vi "Unit test-Encoder triggering.vi"() -> ()   [LabVIEW 2017]
uses:
  Typedefs/Imaging Protocols enum.ctl
  Typedefs/Frame Size.ctl
  Typedefs/Logging queue element.ctl
  Peripherals Control/Pockels/Globals/gl_Pockels control globals.vi
  Typedefs/Acquired points count.ctl
panel:
  out "# of DO points":i32
  in  "Imaging Protocol":T1=enum."Live Imaging"
  out "Waveform Graph":dbl[](graph)
  out "Execution time (ms)":u32
  in  "AO high value":dbl(knob) scale=0.0..2.0
  in  "Start:More:Retriggerable (T)":bool=TRUE
  out "Loop":i32
  out "# of AO points":i32
  in  "stop":bool
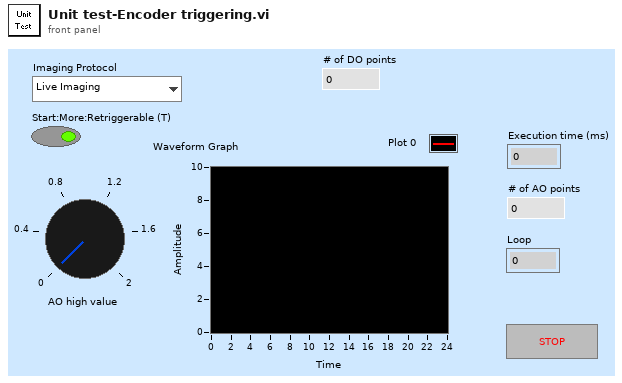
[diagram p1: front panel]
types:
  T1 = typedef "Imaging Protocols enum.ctl" = enum16{"AOL Z-Stack", "Motor Z Stack", "Functional Acquisition", "Single Plane Acquisition", "Volume Acquisition", "Live Imaging", "Live Plane Imaging", "Live Volume Imaging"}
  T2 = typedef "Logging queue element.ctl" = cluster{"Imaging Protocol":T1, "Number of Trials":u16, "Frame Size":T3, "# Averaged frames":u16, "Dwell time (us)":dbl, "Index of Z-plane":i32, "Timelapse?":bool, "Logging process is active":bool, "Speed logging enabled":bool, "tdms file ref":refnum<k34>, "path":path, "Trial Number":i32, "Expected # points acquired":bool, "Manually stopped":bool, "Ch0 data":u32[], "Ch1 data":u32[], "Ref Data":u32[], "Last trial":bool, "Ref Dwell time (us)":dbl, "# Ref Averaged frames":u16, "Ref X Length":u16, "Ref Y Length":u16, "Points acquired":T4}
  T3 = typedef "Frame Size.ctl" = u16
  T4 = typedef "Acquired points count.ctl" = cluster{"Ch0 last trial":u64, "Ch1 last trial":u64, "All trials":u64}
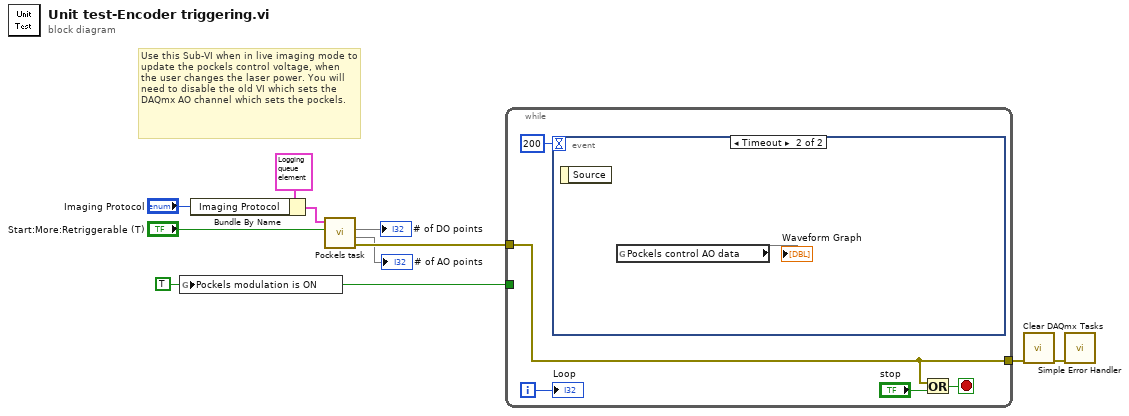
[diagram p0: block diagram]
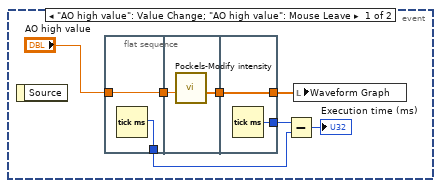
[diagram p2: hidden frame]
diagram:
  w1 = TRUE ("Pockels modulation is ON")
  # "Use this Sub-VI when in live imaging mode to update the pockels control voltage, when the user changes the laser power. You will need to disable the old VI which sets the DAQmx AO channel which sets the pockels."
  n1 = global write "gl_Pockels control globals.vi" "Pockels modulation is ON"(w1) -> ()
  n2 = Bundle By Name(cluster=T2 {"Imaging Protocol"=enum."Live Imaging", "Number of Trials"=0, "Frame Size"=512, "# Averaged frames"=0, "Dwell time (us)"=0.0, "Index of Z-plane"=0, "Timelapse?"=FALSE, "Logging process is active"=FALSE, "Speed logging enabled"=FALSE, "tdms file ref"=refnum, "path"=path "", "Trial Number"=0, "Expected # points acquired"=FALSE, "Manually stopped"=FALSE, "Ch0 data"=[], "Ch1 data"=[], "Ref Data"=[], "Last trial"=FALSE, "Ref Dwell time (us)"=0.0, "# Ref Averaged frames"=0, "Ref X Length"=0, "Ref Y Length"=0, "Points acquired"={"Ch0 last trial"=0, "Ch1 last trial"=0, "All trials"=0}} ("Setup/Logging queue element"), "Imaging Protocol"="Imaging Protocol") -> (w5:T2)
  n3 = call "Pockels task.vi"(10:"Start:More:Retriggerable (T)", "Setup/Logging queue element"=w5) -> ("error out"=w7:errorcluster, 1:→"# of AO points", 2:→"# of DO points")  [unwired: 7 in]
  n4 = while {
    tunnel: w7 -> [w12]
    tunnel: [w12] -> w10
    tunnel: w1 -> [_]
    i -> [w14]
    stop <- w13 stop-if-true
    n5 = event shown="[1] Timeout" {
      selector: _ -> [_ _]
      dyn-events: _ -> [_ _]
      timeout: 200 -> [_ _]
      event "AO high value": Value Change; "AO high value": Mouse Leave {
        n6 = event-data() -> ()  [unwired: 1 in, 1 out]
        n7 = flat-sequence {
          tunnel: "AO high value" -> [w24]
          tunnel: [w24] -> w22
          tunnel: [w23] -> w20
          tunnel: w22 -> [w26]
          tunnel: [w25] -> w18
          tunnel: [w28] -> w21
          tunnel: [w27] -> w17
          tunnel: w18 -> [w27]
          frame #0 {
            n8 = Tick Count (ms)() -> (millisecond timer value=w23:u32)
          }
          frame #1 {
            n9 = call "Pockels-Modify intensity.vi"("Pockels control value (V)"=w26) -> ("Modified data"=w25:dbl[])  [unwired: 9 in, 1 out]
          }
          frame #2 {
            n10 = Tick Count (ms)() -> (millisecond timer value=w28:u32)
          }
        }
        n11 = Subtract(x=w21, y=w20) -> (x-y=→"Execution time (ms)":u32)
        n12 = local write "Waveform Graph"(w17) -> ()
      }
      event Timeout {
        n13 = event-data() -> ()  [unwired: 1 in, 1 out]
        n14 = global read "gl_Pockels control globals.vi" "Pockels control AO data"() -> (→"Waveform Graph")
      }
    }
    n15 = Or(x=w12, y="stop") -> (x .or. y?=w13:bool)
    "Loop" <- w14
  }
  n16 = call "Clear DAQmx Tasks.vi"("error in (no error)"=w10) -> ("error out"=w9:errorcluster)  [unwired: 10 in]
  n17 = call <vilib>:"Simple Error Handler.vi"("error in (no error)"=w9) -> ()  [unwired: 4 in, 5 out]
